vi "Update Microgrid State.vi"(8 "error in":errorcluster, 10 "Microgrid State":T1=enum."Commissioning", 11 "Master Controller in":refnum<class "EMS User Interface.lvclass">) -> (0 "error out":errorcluster, 3 "Master Controller out":refnum<class "EMS User Interface.lvclass">)   [LabVIEW 2018, in "EMS User Interface Actor.lvlib" / "EMS User Interface.lvclass"]
doc: "Sends current state information to front panel."
uses:
  EMS User Interface.lvclass
  EMS Core/EMS/Controls/Microgrid State.ctl
  EMS User Interface.lvclass/EMS User Interface.ctl
  EMS Core/EMS/EMS.lvclass
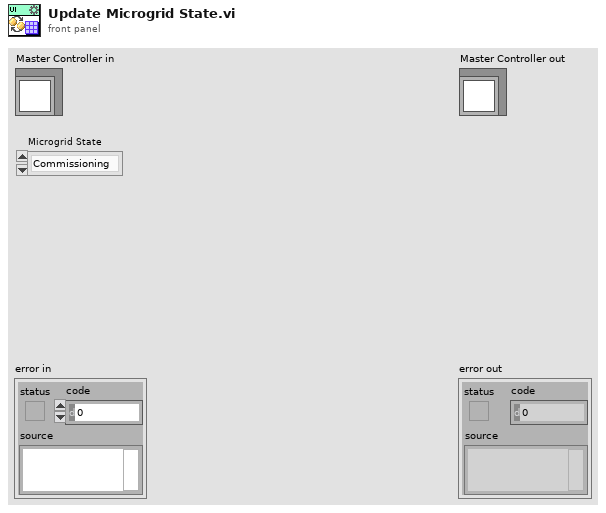
[diagram p1: front panel]
types:
  T1 = typedef "EMS Core.lvlib/EMS.lvclass/Microgrid State.ctl" = enum16{"Discovery", "Commissioning", "Activation", "Blackstart", "OnGrid", "OffGrid", "Island", "Resynchronization", "Manual", "Shutdown", "Stop"}
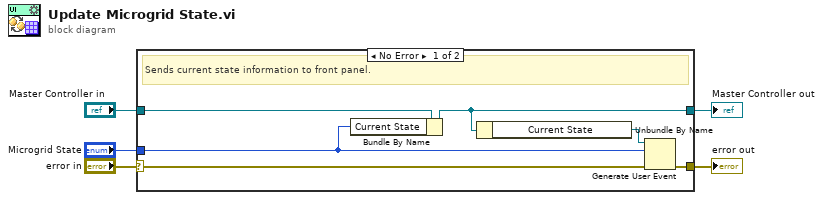
[diagram p0: block diagram]
diagram:
  n1 = case shown="No Error" "error in" {
    selector: "error in" -> [w9 w13]
    tunnel: [w8 w13] -> w4
    tunnel: [w7 w12] -> w2
    tunnel: "Master Controller in" -> [w11 w12]
    tunnel: "Microgrid State" -> [w6 _]
    frame No Error {
      # "Sends current state information to front panel."
      n2 = Bundle By Name(cluster=w11, "Current State"=w6) -> (w7:refnum<class "EMS User Interface.lvclass">)
      n3 = Unbundle By Name(w7) -> ("Current State"=w10:refnum<user-event>)
      n4 = Generate User Event(user event=w10, event data cluster=w6, error in=w9) -> (error out=w8:errorcluster)  [unwired: 1 in, 1 out]
    }
    frame Error {
    }
  }
  "error out" <- w4
  "Master Controller out" <- w2
